vi "Slack-Add To Slack.vi"(0 "client_id":string="1023330033985.1023512746241", 5 "client_secret":string="62f876b60829c507c6cb25bfe9dbba2b") -> (4 "config":T1, 15 "error out":errorcluster)   [LabVIEW 2020]
uses:
  Typedefs/Slack-Configuration.ctl
  <vilib>/Platform/browser.llb/Open URL in Default Browser (string).vi
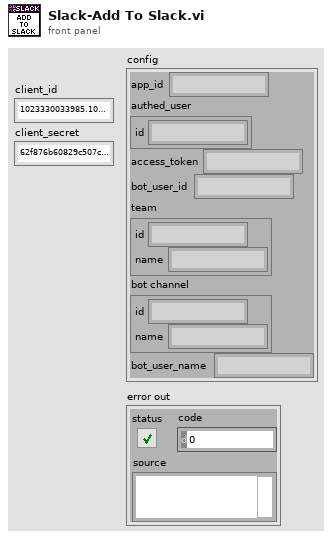
[diagram p1: front panel]
types:
  T1 = typedef "Slack-Configuration.ctl" = cluster{"app_id":string, "authed_user":cluster{"id":string}, "access_token":string, "bot_user_id":string, "team":cluster{"id":string, "name":string}, "bot channel":cluster{"id":string, "name":string}, "bot_user_name":string}
  T2 = typedef "SlackAPI-oauth.v2.access response.ctl" = cluster{"ok":bool, "app_id":string, "authed_user":cluster{"id":string}, "scope":string, "token_type":string, "access_token":string, "bot_user_id":string, "team":cluster{"id":string, "name":string}}
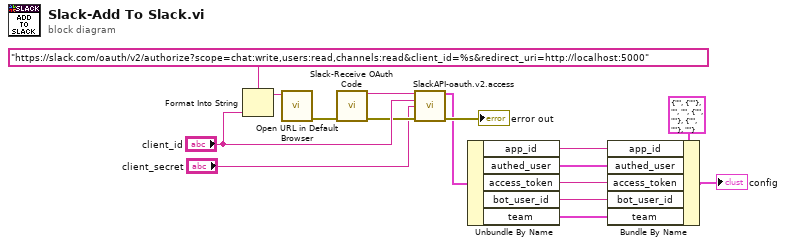
[diagram p0: block diagram]
diagram:
  n1 = Format Into String(format string="https://slack.com/oauth/v2/authorize?scope=chat:write,users:read,channels:read&client_id=%s&redirect_uri=http://localhost:5000", "client_id") -> (resulting string=w14:string)  [unwired: 2 in, 1 out]
  n2 = call-poly <vilib>:"Open URL in Default Browser.vi"("URL"=w14) -> ("error out"=w9:errorcluster)  [unwired: 5 in, 1 out]
  n3 = call "Slack-Receive OAuth Code.vi"("error in (no error)"=w9) -> ("code"=w11:string, "error out"=w13:errorcluster)  [unwired: 13 in]
  n4 = call "SlackAPI-oauth.v2.access.vi"("code"=w11, "client_id"="client_id", "client_secret"="client_secret", "error in (no error)"=w13) -> ("config"=w1:T2, "error out"=→"error out":errorcluster)  [unwired: 10 in]
  n5 = Unbundle By Name(w1) -> ("app_id"=w4:string, "authed_user"=w5:cluster{"id":string}, "access_token"=w6:string, "bot_user_id"=w7:string, "team"=w8:cluster{"id":string, "name":string})
  n6 = Bundle By Name(cluster=T1 {"app_id"="", "authed_user"={"id"=""}, "access_token"="", "bot_user_id"="", "team"={"id"="", "name"=""}, "bot channel"={"id"="", "name"=""}, "bot_user_name"=""} ("Token"), "app_id"=w4, "authed_user"=w5, "access_token"=w6, "bot_user_id"=w7, "team"=w8) -> (→"config":T1)
